vi "dryRun.vi"() -> ()   [LabVIEW 2015]
uses:
  GlobalPath.vi
  GlobalData.vi
  GlobalVi.vi
panel:
  out "PanelName":string
  in  "Done with procedure?":bool
  in  "c-ccd 13":bool caption="Remove stiffback from table"
  in  "Done?":bool
  in  "Open micrometer dry run":bool
  in  "Done gauge?":bool
  in  "Open Gauge Program":bool
  in  "c-ccd 12":bool caption="Position the weights on the stiffback"
  in  "c-ccd 11":bool caption="Release the stiffback from the movement arch"
  in  "c-ccd 10":bool caption="Lower the stiffback on the reference plates"
  in  "c-ccd 9":bool caption="Move the stiffback over the reference plates"
  in  "c-ccd 8":bool caption="Rotate the stiffback upside down"
  in  "c-ccd 7":bool caption="Check cleanliness of the 20 stiffback supports"
  in  "c-ccd 6":bool caption="Mount the 2 stiffback alignment pins on the reference plates"
  # "Dry run preparation"
  # "Dry run tests"
  # "Micrometer measurement of the distance between the reference plates \nand the stiffback plates along the perimeter"
  # "Stiffback surface measurement with gauge system"
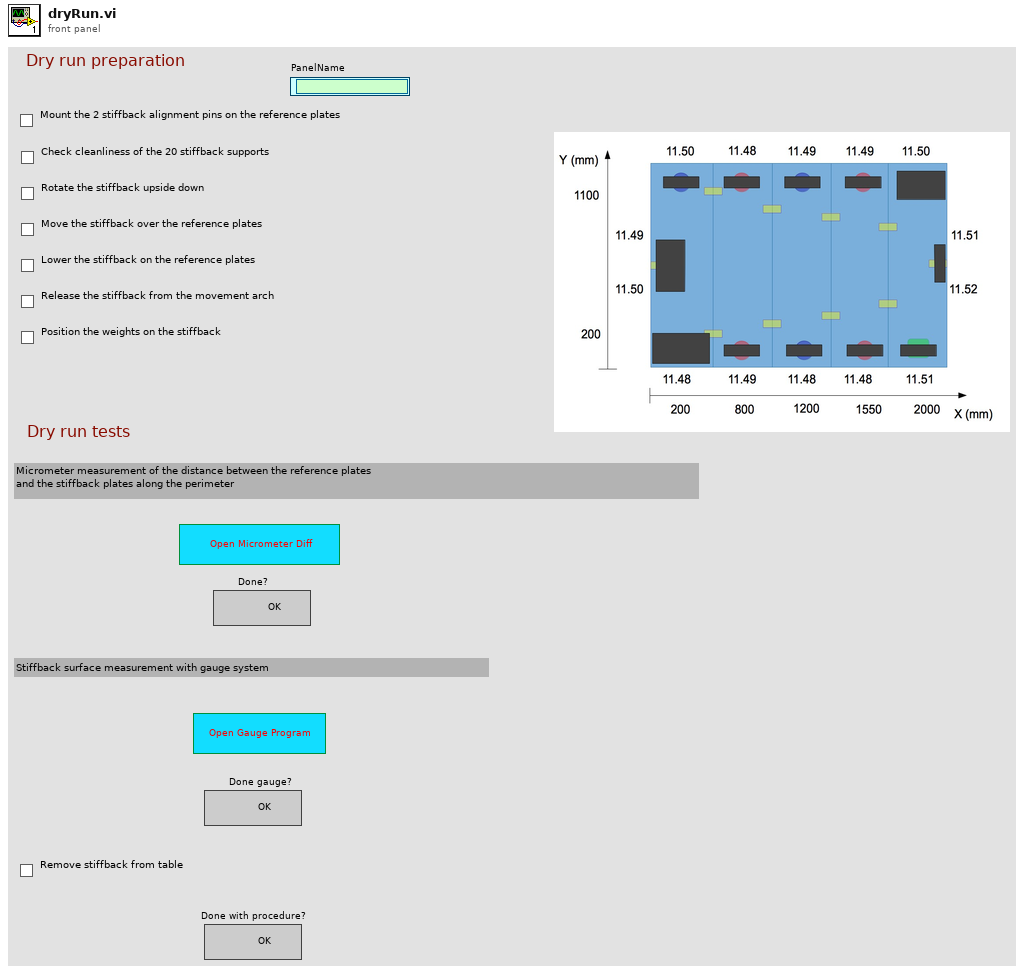
[diagram p1: front panel]
types:
  T1 = enum16{"open", "replace", "create", "open or create", "replace or create", "replace or create with confirmation"}
  T2 = enum32{"Bad", "Idle", "Run top level", "Running"}
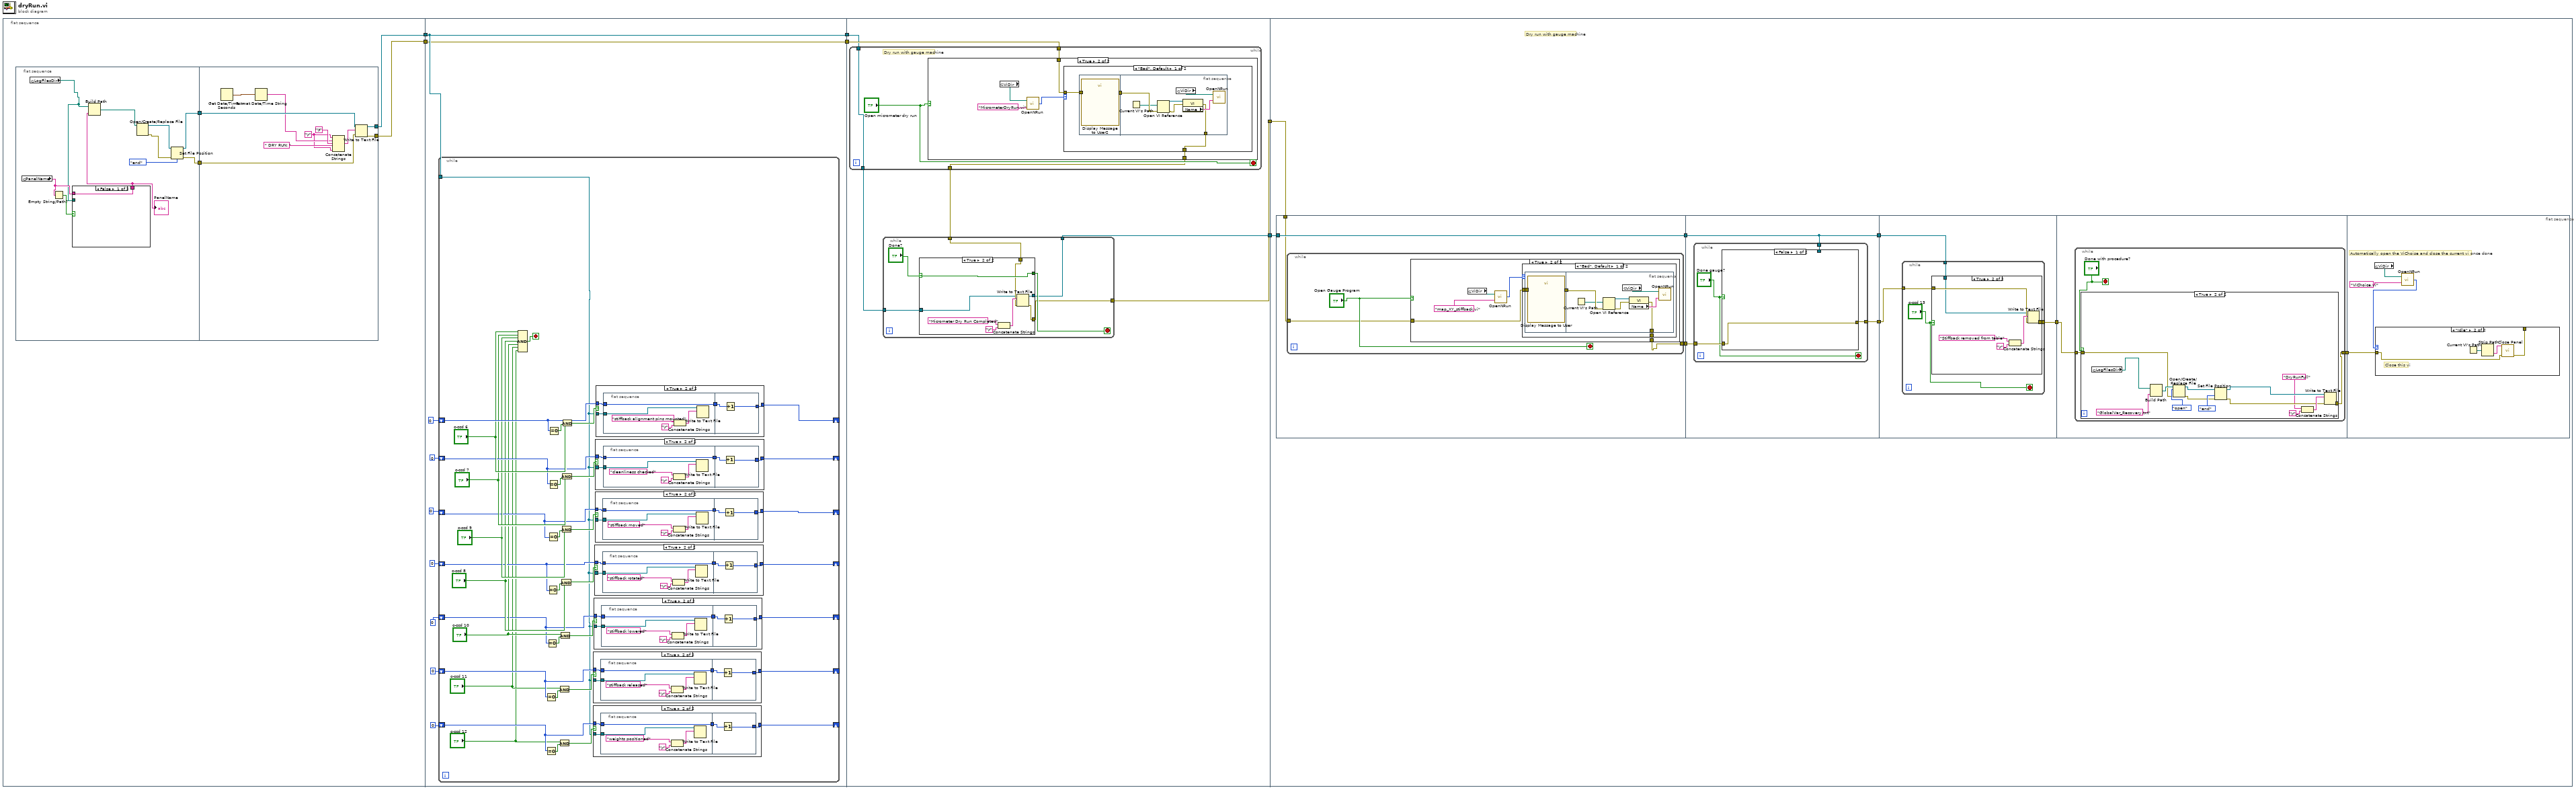
[diagram p0: block diagram]
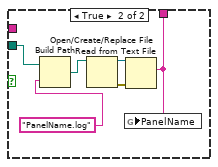
[diagram p2: hidden frame]
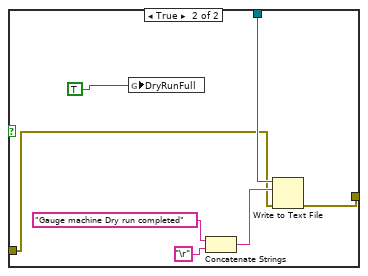
[diagram p15: hidden frame]
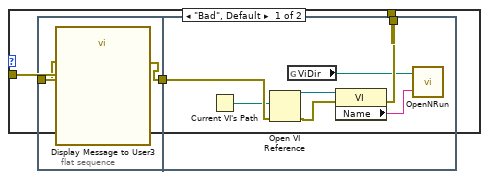
[diagram p18: hidden frame]
diagram:
  n1 = flat-sequence {
    tunnel: [w8] -> w6
    tunnel: [w7] -> w5
    tunnel: w6 -> [w39]
    tunnel: w5 -> [w38]
    tunnel: [w39] -> w4
    tunnel: [w38] -> w3
    tunnel: [w172] -> w2
    tunnel: w4 -> [w170]
    tunnel: w3 -> [w171]
    tunnel: [w168] -> w1
    tunnel: w2 -> [w214]
    tunnel: w1 -> [w219]
    frame #0 {
      n2 = flat-sequence {
        tunnel: [w15] -> w10
        tunnel: [w16] -> w9
        tunnel: w10 -> [w34]
        tunnel: [w33] -> w8
        tunnel: w9 -> [w32]
        tunnel: [w29] -> w7
        frame #0 {
          n3 = global read "GlobalData.vi" "PanelName"() -> (w14:string)
          n4 = global read "GlobalPath.vi" "LogFilesDir"() -> (w12:path)
          n5 = Empty String/Path?(string/path=w14) -> (empty?=w13:bool)
          n6 = case shown="False" w13 {
            tunnel: w12 -> [_ w27]
            tunnel: [w21 w22] -> w11
            tunnel: w14 -> [w21 _]
            frame False {
            }
            frame True {
              n7 = Build Path(base path=w27, name or relative path="PanelName.log") -> (appended path=w26:path)
              n8 = Open/Create/Replace File(file path (use dialog)=w26) -> (refnum out=w23:refnum<file>, error out=w24:errorcluster)  [unwired: 5 in, 1 out]
              n9 = Read from Text File(file (use dialog)=w23, error in=w24) -> (text=w22:string)  [unwired: 2 in, 3 out]
              n10 = global write "GlobalData.vi" "PanelName"(w22) -> ()
            }
          }
          "PanelName" <- w11
          n11 = Build Path(base path=w12, name or relative path=w11) -> (appended path=w20:path)
          n12 = Open/Create/Replace File(file path (use dialog)=w20) -> (refnum out=w18:refnum<file>, error out=w17:errorcluster)  [unwired: 5 in, 1 out]
          n13 = Set File Position(refnum=w18, from (0:start)=enum16{"start", "end", "current"}."end", error in=w17) -> (refnum out=w15:refnum<file>, error out=w16:errorcluster)  [unwired: 1 in]
        }
        frame #1 {
          w28 = "\r"
          n14 = Get Date/Time In Seconds() -> (seconds since 1Jan1904=w31:timestamp)
          n15 = Format Date/Time String(seconds (now)=w31) -> (date/time string=w30:string)  [unwired: 2 in]
          n16 = Concatenate Strings(w28, w30, "\t", " DRY RUN: ", w28) -> (w35:string)
          n17 = Write to Text File(file (use dialog)=w34, text=w35, error in=w32) -> (refnum out=w33:refnum<file>, error out=w29:errorcluster)  [unwired: 1 in, 1 out]
        }
      }
    }
    frame #1 {
      n18 = while {
        tunnel: w39 -> [w48]
        shift-right: [w79] -> _
        shift-left: 0 -> [w81]
        shift-right: [w74] -> _
        shift-left: 0 -> [w76]
        shift-right: [w69] -> _
        shift-left: 0 -> [w70]
        shift-right: [w64] -> _
        shift-left: 0 -> [w65]
        shift-right: [w59] -> _
        shift-left: 0 -> [w60]
        shift-right: [w49] -> _
        shift-left: 0 -> [w53]
        shift-right: [w50] -> _
        shift-left: 0 -> [w54]
        stop <- w47 stop-if-true
        n19 = Compound Arithmetic op=AND("c-ccd 6", "c-ccd 7", "c-ccd 9", "c-ccd 8", "c-ccd 10", "c-ccd 11", "c-ccd 12") -> (w47:bool)
        n20 = Equal To 0?(x=w54) -> (x = 0?=w58:bool)
        n21 = Equal To 0?(x=w53) -> (x = 0?=w56:bool)
        n22 = Equal To 0?(x=w60) -> (x = 0?=w63:bool)
        n23 = Equal To 0?(x=w65) -> (x = 0?=w68:bool)
        n24 = Equal To 0?(x=w70) -> (x = 0?=w73:bool)
        n25 = Equal To 0?(x=w76) -> (x = 0?=w78:bool)
        n26 = Equal To 0?(x=w81) -> (x = 0?=w83:bool)
        n27 = And(x="c-ccd 11", y=w58) -> (x .and. y?=w57:bool)
        n28 = And(x="c-ccd 12", y=w56) -> (x .and. y?=w55:bool)
        n29 = And(x="c-ccd 10", y=w63) -> (x .and. y?=w62:bool)
        n30 = And(x="c-ccd 8", y=w68) -> (x .and. y?=w67:bool)
        n31 = And(x="c-ccd 9", y=w73) -> (x .and. y?=w72:bool)
        n32 = And(x="c-ccd 7", y=w78) -> (x .and. y?=w77:bool)
        n33 = And(x="c-ccd 6", y=w83) -> (x .and. y?=w82:bool)
        n34 = case shown="True" w57 {
          tunnel: w48 -> [_ w100]
          tunnel: w54 -> [w96 w98]
          tunnel: [w96 w97] -> w50
          frame False {
          }
          frame True {
            n35 = flat-sequence {
              tunnel: w100 -> [w102]
              tunnel: [w101] -> w99
              tunnel: w98 -> [w101]
              tunnel: w99 -> [w107]
              tunnel: [w106] -> w97
              frame #0 {
                n36 = Concatenate Strings("stiffback released", "\r") -> (w105:string)
                n37 = Write to Text File(file (use dialog)=w102, text=w105) -> ()  [unwired: 2 in, 3 out]
              }
              frame #1 {
                n38 = Increment(x=w107) -> (x+1=w106:i32)
              }
            }
          }
        }
        n39 = case shown="True" w55 {
          tunnel: w48 -> [_ w88]
          tunnel: w53 -> [w84 w86]
          tunnel: [w84 w85] -> w49
          frame False {
          }
          frame True {
            n40 = flat-sequence {
              tunnel: w88 -> [w90]
              tunnel: [w89] -> w87
              tunnel: w86 -> [w89]
              tunnel: w87 -> [w95]
              tunnel: [w94] -> w85
              frame #0 {
                n41 = Concatenate Strings("weights positioned", "\r") -> (w93:string)
                n42 = Write to Text File(file (use dialog)=w90, text=w93) -> ()  [unwired: 2 in, 3 out]
              }
              frame #1 {
                n43 = Increment(x=w95) -> (x+1=w94:i32)
              }
            }
          }
        }
        n44 = case shown="True" w62 {
          tunnel: w48 -> [_ w112]
          tunnel: w60 -> [w108 w110]
          tunnel: [w108 w109] -> w59
          frame False {
          }
          frame True {
            n45 = flat-sequence {
              tunnel: w112 -> [w114]
              tunnel: [w113] -> w111
              tunnel: w110 -> [w113]
              tunnel: w111 -> [w119]
              tunnel: [w118] -> w109
              frame #0 {
                n46 = Concatenate Strings("stiffback lowered", "\r") -> (w117:string)
                n47 = Write to Text File(file (use dialog)=w114, text=w117) -> ()  [unwired: 2 in, 3 out]
              }
              frame #1 {
                n48 = Increment(x=w119) -> (x+1=w118:i32)
              }
            }
          }
        }
        n49 = case shown="True" w67 {
          tunnel: w48 -> [_ w124]
          tunnel: w65 -> [w120 w122]
          tunnel: [w120 w121] -> w64
          frame False {
          }
          frame True {
            n50 = flat-sequence {
              tunnel: w124 -> [w126]
              tunnel: [w125] -> w123
              tunnel: w122 -> [w125]
              tunnel: w123 -> [w131]
              tunnel: [w130] -> w121
              frame #0 {
                n51 = Concatenate Strings("stiffback rotated", "\r") -> (w129:string)
                n52 = Write to Text File(file (use dialog)=w126, text=w129) -> ()  [unwired: 2 in, 3 out]
              }
              frame #1 {
                n53 = Increment(x=w131) -> (x+1=w130:i32)
              }
            }
          }
        }
        n54 = case shown="True" w72 {
          tunnel: w48 -> [_ w136]
          tunnel: w70 -> [w132 w134]
          tunnel: [w132 w133] -> w69
          frame False {
          }
          frame True {
            n55 = flat-sequence {
              tunnel: w136 -> [w138]
              tunnel: [w137] -> w135
              tunnel: w134 -> [w137]
              tunnel: w135 -> [w143]
              tunnel: [w142] -> w133
              frame #0 {
                n56 = Concatenate Strings("stiffback moved", "\r") -> (w141:string)
                n57 = Write to Text File(file (use dialog)=w138, text=w141) -> ()  [unwired: 2 in, 3 out]
              }
              frame #1 {
                n58 = Increment(x=w143) -> (x+1=w142:i32)
              }
            }
          }
        }
        n59 = case shown="True" w77 {
          tunnel: w48 -> [_ w148]
          tunnel: w76 -> [w144 w146]
          tunnel: [w144 w145] -> w74
          frame False {
          }
          frame True {
            n60 = flat-sequence {
              tunnel: w148 -> [w150]
              tunnel: [w149] -> w147
              tunnel: w146 -> [w149]
              tunnel: w147 -> [w155]
              tunnel: [w154] -> w145
              frame #0 {
                n61 = Concatenate Strings("cleanliness checked", "\r") -> (w153:string)
                n62 = Write to Text File(file (use dialog)=w150, text=w153) -> ()  [unwired: 2 in, 3 out]
              }
              frame #1 {
                n63 = Increment(x=w155) -> (x+1=w154:i32)
              }
            }
          }
        }
        n64 = case shown="True" w82 {
          tunnel: w48 -> [_ w160]
          tunnel: w81 -> [w156 w158]
          tunnel: [w156 w157] -> w79
          frame False {
          }
          frame True {
            n65 = flat-sequence {
              tunnel: w160 -> [w162]
              tunnel: [w161] -> w159
              tunnel: w158 -> [w161]
              tunnel: w159 -> [w167]
              tunnel: [w166] -> w157
              frame #0 {
                n66 = Concatenate Strings("stiffback alignment pins mounted", "\r") -> (w165:string)
                n67 = Write to Text File(file (use dialog)=w162, text=w165) -> ()  [unwired: 2 in, 3 out]
              }
              frame #1 {
                n68 = Increment(x=w167) -> (x+1=w166:i32)
              }
            }
          }
        }
      }
    }
    frame #2 {
      n69 = while {
        tunnel: [w174] -> w173
        tunnel: w171 -> [w177]
        tunnel: [w176] -> w169
        tunnel: w170 -> [w176]
        stop <- "Open micrometer dry run" stop-if-true
        # "Dry run with gauge machine"
        n70 = case shown="True" "Open micrometer dry run" {
          tunnel: w177 -> [w178 w183]
          tunnel: [w178 w182] -> w174
          frame False {
          }
          frame True {
            n71 = global read "GlobalPath.vi" "ViDir"() -> (w181:path)
            n72 = call "OpenNRun.vi"("VI name"="MicrometerDryRun.vi", "ViDirPath"=w181) -> ("Execution:State"=w180:T2)
            n73 = case shown="\"Bad\", Default" w180 {
              tunnel: [w185 _] -> w182
              tunnel: w183 -> [w184 _]
              frame "Bad", Default {
                n74 = flat-sequence {
                  tunnel: [w188] -> w186
                  tunnel: w184 -> [w187]
                  tunnel: w186 -> [w191]
                  tunnel: [w190] -> w185
                  frame #0 {
                    n75 = call "Display Message to User2"("error in (no error)"=w187) -> ("error out"=w188:errorcluster)  [unwired: 9 in, 1 out]
                  }
                  frame #1 {
                    n76 = Current VI's Path() -> (path=w189:path)
                    n77 = Open VI Reference(vi path=w189, error in (no error)=w191) -> (vi reference=w195:refnum<vi>, error out=w194:errorcluster)  [unwired: 4 in]
                    n78 = global read "GlobalPath.vi" "ViDir"() -> (w193:path)
                    n79 = property class="VI"(reference=w195, error in=w194) -> (error out=w190:errorcluster, "Name"=w192:string)  [unwired: 1 out]
                    n80 = call "OpenNRun.vi"("VI name"=w192, "ViDirPath"=w193) -> ()  [unwired: 1 out]
                  }
                }
              }
              frame "Idle" {
              }
            }
          }
        }
      }
      n81 = while {
        tunnel: w173 -> [w199]
        tunnel: [w198] -> w172
        tunnel: w169 -> [w197]
        tunnel: [w196] -> w168
        stop <- w201 stop-if-true
        n82 = case shown="True" "Done?" {
          selector: "Done?" -> [w204 w209]
          tunnel: [w204 w209] -> w201
          tunnel: w199 -> [w203 w208]
          tunnel: [w203 w207] -> w198
          tunnel: w197 -> [w202 w206]
          tunnel: [w202 w205] -> w196
          frame False {
          }
          frame True {
            n83 = Concatenate Strings("Micrometer Dry Run Completed", "\r") -> (w212:string)
            n84 = Write to Text File(file (use dialog)=w206, text=w212, error in=w208) -> (refnum out=w205:refnum<file>, error out=w207:errorcluster)  [unwired: 1 in, 1 out]
          }
        }
      }
    }
    frame #3 {
      # "Dry run with gauge machine"
      n85 = flat-sequence {
        tunnel: w219 -> [w223]
        tunnel: [w223] -> w215
        tunnel: w214 -> [w222]
        tunnel: [w221] -> w213
        tunnel: [w248] -> w218
        tunnel: [w247] -> w217
        tunnel: w215 -> [w248]
        tunnel: w213 -> [w246]
        tunnel: w218 -> [w263]
        tunnel: w217 -> [w262]
        tunnel: [w261] -> w216
        tunnel: [w276] -> w220
        tunnel: w216 -> [w275]
        tunnel: w220 -> [w295]
        frame #0 {
          n86 = while {
            tunnel: w222 -> [w225]
            tunnel: [w224] -> w221
            stop <- "Open Gauge Program" stop-if-true
            n87 = case shown="True" "Open Gauge Program" {
              tunnel: [w227 w230] -> w224
              tunnel: w225 -> [w227 w229]
              frame False {
              }
              frame True {
                n88 = global read "GlobalPath.vi" "ViDir"() -> (w232:path)
                n89 = call "OpenNRun.vi"("VI name"="map_XY_stiffback.vi", "ViDirPath"=w232) -> ("Execution:State"=w231:T2)
                n90 = case shown="\"Bad\", Default" w231 {
                  tunnel: [w234 w245] -> w230
                  tunnel: w229 -> [w233 w245]
                  frame "Bad", Default {
                    n91 = flat-sequence {
                      tunnel: [w236] -> w235
                      tunnel: w233 -> [w237]
                      tunnel: w235 -> [w240]
                      tunnel: [w239] -> w234
                      frame #0 {
                        n92 = call "Display Message to User"("error in (no error)"=w237) -> ("error out"=w236:errorcluster)  [unwired: 9 in, 1 out]
                      }
                      frame #1 {
                        n93 = Current VI's Path() -> (path=w238:path)
                        n94 = Open VI Reference(vi path=w238, error in (no error)=w240) -> (vi reference=w244:refnum<vi>, error out=w243:errorcluster)  [unwired: 4 in]
                        n95 = global read "GlobalPath.vi" "ViDir"() -> (w242:path)
                        n96 = property class="VI"(reference=w244, error in=w243) -> (error out=w239:errorcluster, "Name"=w241:string)  [unwired: 1 out]
                        n97 = call "OpenNRun.vi"("VI name"=w241, "ViDirPath"=w242) -> ()  [unwired: 1 out]
                      }
                    }
                  }
                  frame "Idle" {
                  }
                }
              }
            }
          }
        }
        frame #1 {
          n98 = while {
            tunnel: w248 -> [w252]
            tunnel: [w251] -> w247
            tunnel: w246 -> [w250]
            stop <- "Done gauge?" stop-if-true
            n99 = case shown="False" "Done gauge?" {
              tunnel: [w253 w257] -> w251
              tunnel: w252 -> [_ w255]
              tunnel: w250 -> [w253 w254]
              frame False {
              }
              frame True {
                n100 = global write "GlobalVi.vi" "DryRunFull"(TRUE) -> ()
                n101 = Concatenate Strings("Gauge machine Dry run completed", "\r") -> (w260:string)
                n102 = Write to Text File(file (use dialog)=w255, text=w260, error in=w254) -> (error out=w257:errorcluster)  [unwired: 1 in, 2 out]
              }
            }
          }
        }
        frame #2 {
          n103 = while {
            tunnel: w262 -> [w267]
            tunnel: w263 -> [w266]
            tunnel: [w265] -> w261
            stop <- "c-ccd 13" stop-if-true
            n104 = case shown="True" "c-ccd 13" {
              tunnel: w267 -> [w268 w271]
              tunnel: w266 -> [_ w270]
              tunnel: [w268 w269] -> w265
              frame False {
              }
              frame True {
                n105 = Concatenate Strings("Stiffback removed from table", "\r") -> (w274:string)
                n106 = Write to Text File(file (use dialog)=w270, text=w274, error in=w271) -> (error out=w269:errorcluster)  [unwired: 1 in, 2 out]
              }
            }
          }
        }
        frame #3 {
          n107 = while {
            tunnel: w275 -> [w278]
            tunnel: [w279] -> w276
            stop <- "Done with procedure?" stop-if-true
            n108 = case shown="True" "Done with procedure?" {
              tunnel: [w280 w284] -> w279
              tunnel: w278 -> [w280 w282]
              frame False {
              }
              frame True {
                n109 = global read "GlobalPath.vi" "LogFilesDir"() -> (w281:path)
                n110 = Build Path(base path=w281, name or relative path="GlobalVar_Recovery.txt") -> (appended path=w293:path)
                n111 = Open/Create/Replace File(file path (use dialog)=w293, error in=w282, operation (0:open)=T1."open") -> (refnum out=w289:refnum<file>, error out=w290:errorcluster)  [unwired: 3 in, 1 out]
                n112 = Set File Position(refnum=w289, from (0:start)=enum16{"start", "end", "current"}."end", error in=w290) -> (refnum out=w286:refnum<file>, error out=w285:errorcluster)  [unwired: 1 in]
                n113 = Concatenate Strings("DryRunFull", "\r") -> (w288:string)
                n114 = Write to Text File(file (use dialog)=w286, text=w288, error in=w285) -> (error out=w284:errorcluster)  [unwired: 1 in, 2 out]
              }
            }
          }
        }
        frame #4 {
          # "Automatically open the ViChoise and close the current vi once done"
          n115 = global read "GlobalPath.vi" "ViDir"() -> (w298:path)
          n116 = call "OpenNRun.vi"("VI name"="ViChoice.vi", "ViDirPath"=w298) -> ("Execution:State"=w297:T2)
          n117 = case shown="\"Idle\"" w297 {
            tunnel: [w301 w311] -> _
            tunnel: w295 -> [w300 w312]
            frame "Bad", Default {
              n118 = flat-sequence {
                tunnel: w300 -> [w303]
                tunnel: [w302] -> w299
                tunnel: [w307] -> w301
                tunnel: w299 -> [w306]
                frame #0 {
                  n119 = call "Display Message to User3"("error in (no error)"=w303) -> ("error out"=w302:errorcluster)  [unwired: 9 in, 1 out]
                }
                frame #1 {
                  n120 = Current VI's Path() -> (path=w304:path)
                  n121 = Open VI Reference(vi path=w304, error in (no error)=w306) -> (vi reference=w310:refnum<vi>, error out=w309:errorcluster)  [unwired: 4 in]
                  n122 = global read "GlobalPath.vi" "ViDir"() -> (w305:path)
                  n123 = property class="VI"(reference=w310, error in=w309) -> (error out=w307:errorcluster, "Name"=w308:string)  [unwired: 1 out]
                  n124 = call "OpenNRun.vi"("VI name"=w308, "ViDirPath"=w305) -> ()  [unwired: 1 out]
                }
              }
            }
            frame "Idle" {
              # "Close this vi"
              n125 = Current VI's Path() -> (path=w314:path)
              n126 = Strip Path(path=w314) -> (name=w313:string)  [unwired: 1 out]
              n127 = call <vilib>:"Close Panel.vi"("error in (no error)"=w312, "VI name"=w313) -> ("error out"=w311:errorcluster)  [unwired: 9 in]
            }
          }
        }
      }
    }
  }
